vi "Initialize.vi"(8 "error in":errorcluster, 11 "TCP master in":refnum<class "SMSD Master.lvclass">) -> (0 "error out":errorcluster, 3 "TCP master out":refnum<class "SMSD Master.lvclass">)   [LabVIEW 2021, in "SMSD Master.lvclass"]
doc: "Opens a TCP connection to the address and port stored in the class."
uses:
  SMSD Master.lvclass
  SMSD Master.lvclass/SMSD Master.ctl
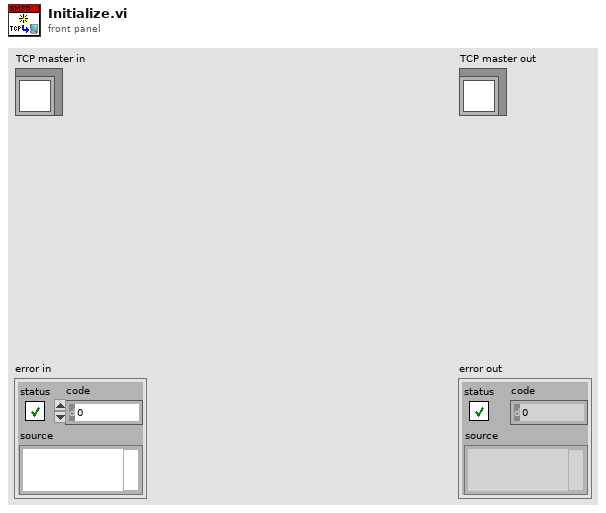
[diagram p1: front panel]
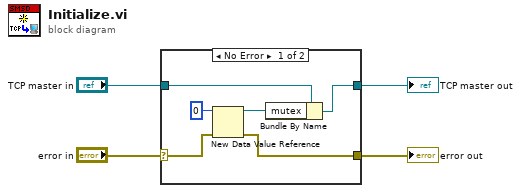
[diagram p0: block diagram]
diagram:
  n1 = case shown="No Error" "error in" {
    selector: "error in" -> [w5 w12]
    tunnel: "TCP master in" -> [w8 w11]
    tunnel: [w7 w11] -> w2
    tunnel: [w6 w12] -> w1
    frame No Error {
      n2 = New Data Value Reference(data value=u8 0, error in=w5) -> (data value reference=w9:refnum<data-value>, error out=w6:errorcluster)
      n3 = Bundle By Name(cluster=w8, "mutex"=w9) -> (w7:refnum<class "SMSD Master.lvclass">)
    }
    frame Error {
    }
  }
  "error out" <- w1
  "TCP master out" <- w2
